vi "3D Offset Object Z.vi"(7 "Offset":dbl, 8 "Scene:New Object":refnum<vi>) -> (2 "Scene.Object Out":refnum<vi>)   [LabVIEW 2017]
uses:
  <vilib>/picture/3D Picture Control/NI_3D Picture Control.lvlib
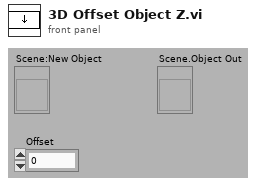
[diagram p1: front panel]
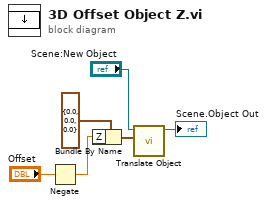
[diagram p0: block diagram]
diagram:
  n1 = Negate(x="Offset") -> (-x=w1:dbl)
  n2 = Bundle By Name(cluster=cluster{"X":sgl, "Y":sgl, "Z":sgl} {"X"=0.0, "Y"=0.0, "Z"=0.0} ("Translation"), "Z"=w1) -> (w4:cluster{"X":sgl, "Y":sgl, "Z":sgl})
  n3 = call <vilib>:"Translate Object.vi"("Translation"=w4, "Scene.Object In"="Scene:New Object") -> ("Scene.Object Out"=→"Scene.Object Out":refnum<vi>)  [unwired: 1 in, 8 out]
